vi "Actor Core.vi"(8 "Error In":errorcluster, 11 "LHW-GUI-Actor in":refnum<class "LHW-GUI-Actor.lvclass">) -> (0 "Error Out":errorcluster, 3 "Actor out":refnum<class "Actor.lvclass">)   [LabVIEW 2014, in "LHW-GUI.lvlib" / "LHW-GUI-Actor.lvclass"]
doc: "(<B>Filename</B>: Actor Framework.lvlib:Actor.lvclass:Actor Core.vi)\n\nReceives messages to the actor, reacts to them, and initiates any error handling that may shut the actor down.\n\nDescendant classes may override this VI to append parallel tasks for the actor to complete while it handles messages. Overrides use the Call Parent Method node."
uses:
  LHW-GUI-Actor.lvclass
  <vilib>/ActorFramework/Actor/Actor.lvclass
  Classes/LHW-Data/LHW-Data/LHW-Data.lvclass
  LHW-GUI-Actor.lvclass/LHW-GUI-Actor.ctl
  <vilib>/ActorFramework/Actor/Actor.lvclass/Actor.ctl
  <vilib>/ActorFramework/Message Enqueuer/Message Enqueuer.lvclass/Message Enqueuer.ctl
  LHW-DataGenerator/LHW-GenerateData/LHW-DataGenerator-Actor.lvclass
  LHW-Storage/LHW-Analysis-Actor.lvclass
  LHW-TDMS-Storage/LHW-TDMS-Storage-Actor.lvclass
  LHW-GUI-Actor Messages/Launch Nested Actors Msg/Launch Nested Actors Msg.lvclass/Launch Nested Actors Msg.ctl
  LHW-GUI-Actor Messages/Start-Stop DAQ Msg/Start-Stop DAQ Msg.lvclass/Start-Stop DAQ Msg.ctl
  Classes/LHW-Data/LHW-WfmData/LHW-WfmData.lvclass
  Classes/LHW-Data/LHW-Data/LHW-Data.lvclass/LHW-Data.ctl
  Classes/LHW-Data/LHW-WfmData/LHW-WfmData.lvclass/LHW-WfmData.ctl
  Classes/LHW-Data/LHW-Data/Read Error.vi
  Classes/LHW-Data/LHW-WfmData/Read Waveform Array.vi
  <vilib>/ActorFramework/Message Enqueuer/Init from Existing Queue.vi
  <vilib>/ActorFramework/Message Enqueuer/Enqueue.vi
  <vilib>/ActorFramework/Message Priority Queue/Priority Enqueue.vi
  <vilib>/ActorFramework/Message Enqueuer/Message Enqueuer.lvclass
  <vilib>/ActorFramework/Stop Msg/Stop Msg.lvclass
  LHW-GUI-Actor Messages/Launch Nested Actors Msg/Launch Nested Actors Msg.lvclass
  LHW-GUI-Actor Messages/Stop Nested Actors Msg/Stop Nested Actors Msg.lvclass
  LHW-GUI-Actor Messages/Start-Stop DAQ Msg/Start-Stop DAQ Msg.lvclass
panel:
  out "Waveform Graph":waveform(dbl)[](graph)
  out "DAQ Active":bool
  in  "Start DAQ":bool
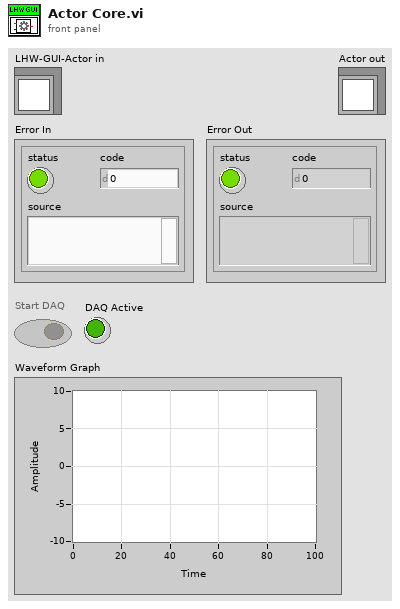
[diagram p1: front panel]
types:
  T1 = enum8{"Enabled", "Disabled", "Disabled and Grayed Out"}
  T2 = cluster{"LHW-Aquisition-Actor":refnum<class "LHW-DataGenerator-Actor.lvclass">, "LHW-Analysis-Actor":refnum<class "LHW-Analysis-Actor.lvclass">, "LHW-Storage-Actor":refnum<class "LHW-TDMS-Storage-Actor.lvclass">}
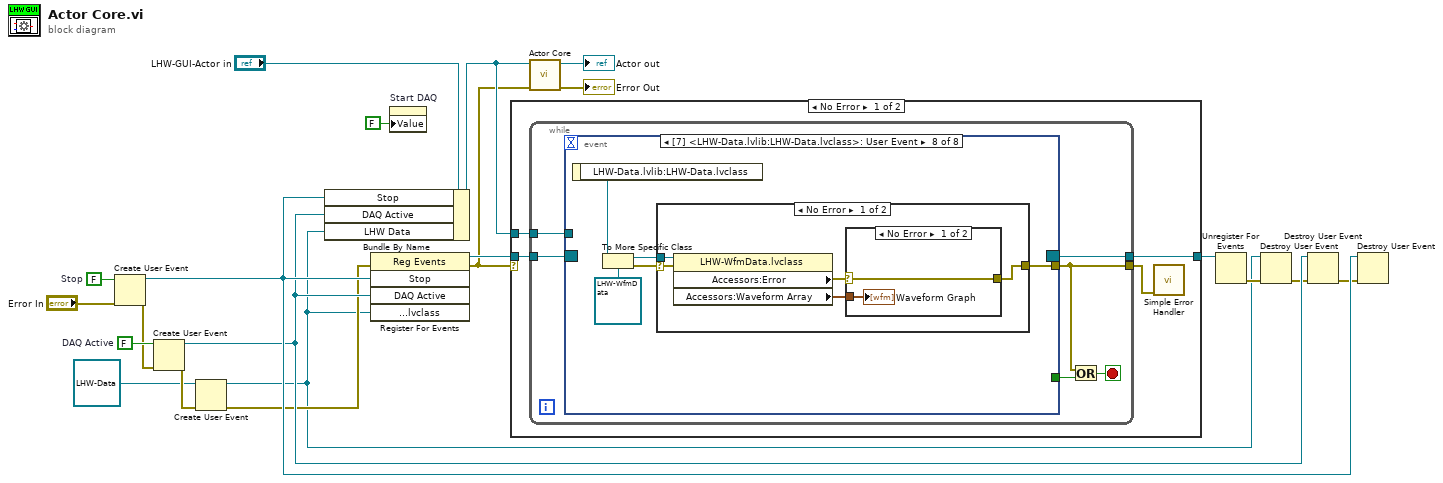
[diagram p0: block diagram]
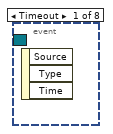
[diagram p2: hidden frame]
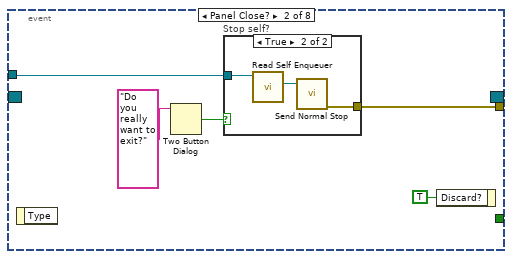
[diagram p3: hidden frame]
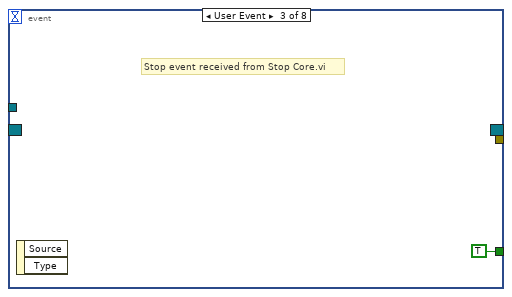
[diagram p5: hidden frame]
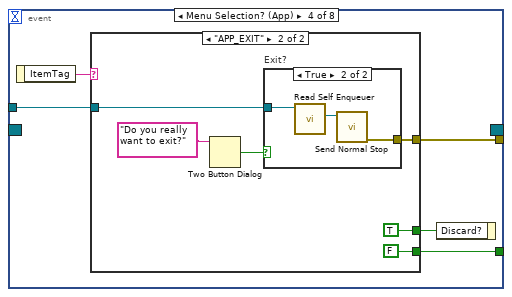
[diagram p6: hidden frame]
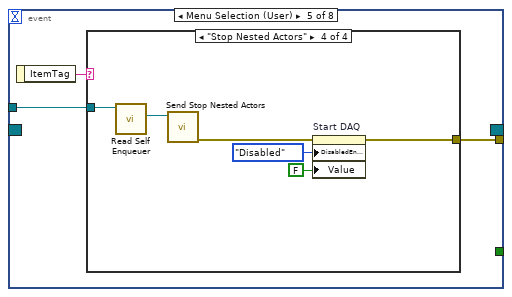
[diagram p9: hidden frame]
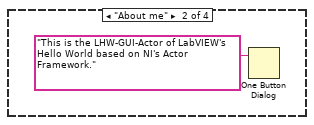
[diagram p11: hidden frame]
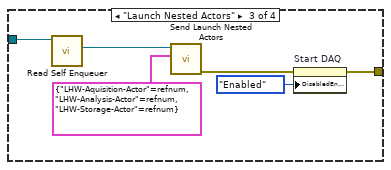
[diagram p12: hidden frame]
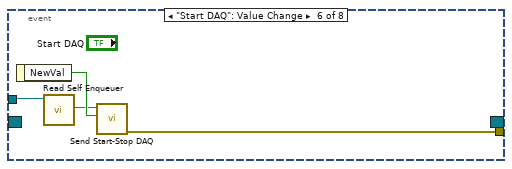
[diagram p13: hidden frame]
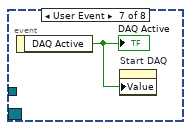
[diagram p14: hidden frame]
diagram:
  w11 = FALSE  # DAQ Active
  w19 = FALSE  # Stop
  n1 = Create User Event(user event datatype=w19, error in="Error In") -> (user event=w12:refnum<user-event>, error out=w10:errorcluster)
  n2 = Create User Event(user event datatype=w11, error in=w10) -> (user event=w8:refnum<user-event>, error out=w6:errorcluster)
  n3 = Create User Event(user event datatype=refnum<class "LHW-Data.lvclass"> refnum ("LHW-Data.lvlib:LHW-Data.lvclass"), error in=w6) -> (user event=w1:refnum<user-event>, error out=w5:errorcluster)
  n4 = Bundle By Name(cluster="LHW-GUI-Actor in", "Stop"=w12, "DAQ Active"=w8, "LHW Data"=w1) -> (w16:refnum<class "LHW-GUI-Actor.lvclass">)
  n5 = register-events(error in=w5, w12, w8, w1) -> (reference out=w18:refnum<event-registration>, error out=w14:errorcluster)  [unwired: 1 in]
  n6 = property on="Start DAQ" class="Bool (strict)"("Value"=FALSE ("Start DAQ")) -> ()  [unwired: 2 in, 2 out]
  n7 = case shown="No Error" w14 {
    tunnel: w18 -> [w25 w90]
    tunnel: w16 -> [w24 _]
    tunnel: [w23 w90] -> w13
    frame No Error {
      n8 = while {
        tunnel: [w29] -> w22
        tunnel: w24 -> [w28]
        tunnel: w25 -> [w27]
        tunnel: [w26] -> w23
        stop <- w30 stop-if-true
        n9 = event shown="[7] <LHW-Data.lvlib:LHW-Data.lvclass>: User Event" {
          selector: w27 -> [_ _ _ _ _ _ _ _]
          dyn-events: [_ _ _ _ _ _ _ _] -> w26
          timeout: _ -> [_ _ _ _ _ _ _ _]
          tunnel: [_ w33 _ w43 w55 w73 _ w77] -> w29
          tunnel: [_ _ TRUE ("T button?") w45 _ _ _ _] -> w31
          tunnel: w28 -> [_ w32 _ w41 w56 w74 _ _]
          event Timeout {
            n10 = event-data() -> ()  [unwired: 1 in, 3 out]
          }
          event Panel Close? {
            n11 = event-data() -> ()  [unwired: 1 in, 1 out]
            n12 = Two Button Dialog(message="Do you really want to exit?") -> (T button?=w35:bool)  [unwired: 2 in]
            n13 = case "Stop self?" shown="True" w35 {
              tunnel: [_ w39] -> w33
              tunnel: w32 -> [_ w37]
              frame False {
              }
              frame True {
                n14 = call <vilib>:"Read Self Enqueuer.vi"("Actor"=w37) -> ("Self Enqueuer"=w38:refnum<class "Message Enqueuer.lvclass">)  [unwired: 10 in]
                n15 = call <vilib>:"Send Normal Stop.vi"("Message Enqueuer"=w38) -> ("error out"=w39:errorcluster)  [unwired: 10 in]
              }
            }
            n16 = event-data("Discard?"=TRUE) -> ()  [unwired: 1 in, 1 out]
          }
          event User Event {
            # "Stop event received from Stop Core.vi"
            n17 = event-data() -> ()  [unwired: 1 in, 2 out]
          }
          event Menu Selection? (App) {
            n18 = event-data() -> ("ItemTag"=w44:string)  [unwired: 1 in]
            n19 = case shown="\"APP_EXIT\"" w44 {
              tunnel: [_ FALSE ("T button?")] -> w45
              tunnel: [_ w49] -> w43
              tunnel: [_ TRUE ("Discard?")] -> w42
              tunnel: w41 -> [_ w47]
              frame Default {
              }
              frame "APP_EXIT" {
                n20 = Two Button Dialog(message="Do you really want to exit?") -> (T button?=w51:bool)  [unwired: 2 in]
                n21 = case "Exit?" shown="True" w51 {
                  tunnel: [_ w54] -> w49
                  tunnel: w47 -> [_ w52]
                  frame False {
                  }
                  frame True {
                    n22 = call <vilib>:"Read Self Enqueuer.vi"("Actor"=w52) -> ("Self Enqueuer"=w53:refnum<class "Message Enqueuer.lvclass">)  [unwired: 10 in]
                    n23 = call <vilib>:"Send Normal Stop.vi"("Message Enqueuer"=w53) -> ("error out"=w54:errorcluster)  [unwired: 10 in]
                  }
                }
              }
            }
            n24 = event-data("Discard?"=w42) -> ()  [unwired: 1 in, 1 out]
          }
          event Menu Selection (User) {
            n25 = event-data() -> ("ItemTag"=w57:string)  [unwired: 1 in]
            n26 = case shown="\"Stop Nested Actors\"" w57 {
              tunnel: w56 -> [_ _ w64 w70]
              tunnel: [_ _ w59 w66] -> w55
              frame Default {
              }
              frame "About me" {
                n27 = One Button Dialog(message="This is the LHW-GUI-Actor of LabVIEW's Hello World based on NI's Actor Framework.") -> ()  [unwired: 1 in, 1 out]
              }
              frame "Launch Nested Actors" {
                n28 = call <vilib>:"Read Self Enqueuer.vi"("Actor"=w64) -> ("Self Enqueuer"=w63:refnum<class "Message Enqueuer.lvclass">)  [unwired: 10 in]
                n29 = call "Send Launch Nested Actors.vi"("Nested Actors"=T2 {"LHW-Aquisition-Actor"=refnum, "LHW-Analysis-Actor"=refnum, "LHW-Storage-Actor"=refnum}, "Message Enqueuer"=w63) -> ("error out"=w60:errorcluster)  [unwired: 8 in, 1 out]
                n30 = property on="Start DAQ" class="Bool (strict)"(error in=w60, "DisabledEnum"=T1."Enabled" ("Disabled")) -> (error out=w59:errorcluster)  [unwired: 1 in, 1 out]
              }
              frame "Stop Nested Actors" {
                n31 = call <vilib>:"Read Self Enqueuer.vi"("Actor"=w70) -> ("Self Enqueuer"=w69:refnum<class "Message Enqueuer.lvclass">)  [unwired: 10 in]
                n32 = call "Send Stop Nested Actors.vi"("Message Enqueuer"=w69) -> ("error out"=w67:errorcluster)  [unwired: 9 in, 1 out]
                n33 = property on="Start DAQ" class="Bool (strict)"(error in=w67, "DisabledEnum"=T1."Disabled" ("Disabled"), "Value"=FALSE ("Start DAQ")) -> (error out=w66:errorcluster)  [unwired: 1 in, 1 out]
              }
            }
          }
          event "Start DAQ": Value Change {
            n34 = event-data() -> ("NewVal"=w72:bool)  [unwired: 1 in]
            n35 = call <vilib>:"Read Self Enqueuer.vi"("Actor"=w74) -> ("Self Enqueuer"=w71:refnum<class "Message Enqueuer.lvclass">)  [unwired: 10 in]
            n36 = call "Send Start-Stop DAQ.vi"("Start DAQ"=w72, "Message Enqueuer"=w71) -> ("error out"=w73:errorcluster)  [unwired: 8 in, 1 out]
          }
          event User Event {
            n37 = event-data() -> ("DAQ Active"=w75:bool)  [unwired: 1 in]
            "DAQ Active" <- w75
            n38 = property on="Start DAQ" class="Bool (strict)"("Value"=w75) -> ()  [unwired: 2 in, 2 out]
          }
          event User Event {
            n39 = event-data() -> ("LHW-Data.lvlib:LHW-Data.lvclass"=w80:refnum<class "LHW-Data.lvclass">)  [unwired: 1 in]
            n40 = To More Specific Class(target class=refnum<class "LHW-WfmData.lvclass"> refnum ("LHW-Data.lvlib:LHW-WfmData.lvclass"), reference=w80) -> (specific class reference=w76:refnum<class "LHW-WfmData.lvclass">, error out=w78:errorcluster)  [unwired: 1 in]
            n41 = case shown="No Error" w78 {
              selector: w78 -> [w82 w89]
              tunnel: [w81 w89] -> w77
              tunnel: w76 -> [w85 _]
              frame No Error {
                n42 = property class="LHW-WfmData.lvclass"(reference=w85, error in=w82) -> ("Accessors:Error"=w84:errorcluster, "Accessors:Waveform Array"=w83:waveform(dbl)[])  [unwired: 2 out]
                n43 = case shown="No Error" w84 {
                  selector: w84 -> [w86 w88]
                  tunnel: w83 -> [w87 _]
                  tunnel: [w86 w88] -> w81
                  frame No Error {
                    "Waveform Graph" <- w87
                  }
                  frame Error {
                  }
                }
              }
              frame Error {
              }
            }
          }
        }
        n44 = Or(x=w29, y=w31) -> (x .or. y?=w30:bool)
      }
      n45 = call <vilib>:"Simple Error Handler.vi"("error in (no error)"=w22) -> ()  [unwired: 4 in, 5 out]
    }
    frame Error {
    }
  }
  n46 = call-parent "Actor Core.vi"("error in"=w14, "Actor in"=w16) -> ("error out"=→"Error Out":errorcluster, "Actor out"=→"Actor out":refnum<class "Actor.lvclass">)  [unwired: 8 in]
  n47 = Unregister For Events(event registration refnum=w13) -> (error out=w3:errorcluster)  [unwired: 1 in]
  n48 = Destroy User Event(user event=w1, error in=w3) -> (error out=w2:errorcluster)
  n49 = Destroy User Event(user event=w8, error in=w2) -> (error out=w9:errorcluster)
  n50 = Destroy User Event(user event=w12, error in=w9) -> ()  [unwired: 1 out]
